vi "ReadKeithley6485Configuration.vi"(8 "Error In":errorcluster, 11 "ABLE Config File Ref In":T2) -> (0 "Error Out":errorcluster, 2 "Keithley 6485 Configuration":T1, 3 "ABLE Config File Ref Out":T2)   [LabVIEW 2012]
uses:
  <vilib>/Utility/config.llb/Config Data RefNum.ctl
  Keithley6485Configuration.ctl
  <vilib>/Utility/config.llb/Read Key (String).vi
  <vilib>/Utility/config.llb/NI_LVConfig.lvlib
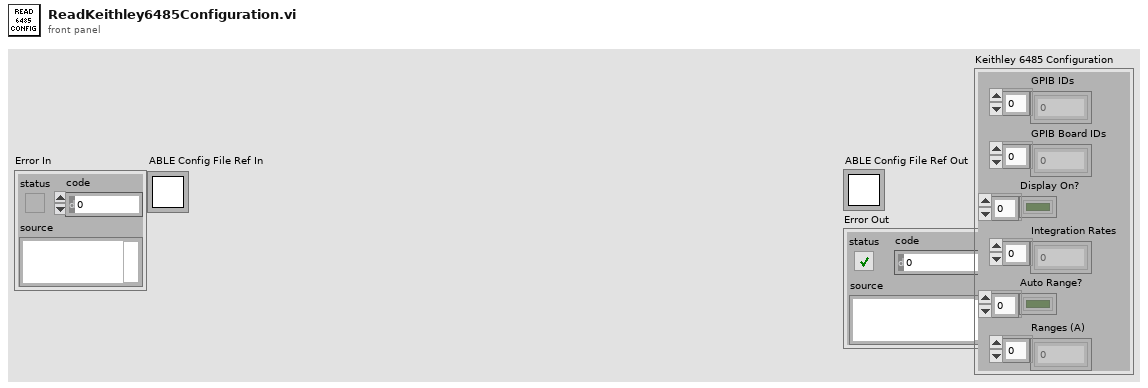
[diagram p1: front panel]
types:
  T1 = typedef "Keithley6485Configuration.ctl" = cluster{"GPIB IDs":u8[], "GPIB Board IDs":u8[], "Display On?":bool[], "Integration Rates":dbl[], "Auto Range?":bool[], "Ranges (A)":dbl[]}
  T2 = typedef "NI_LVConfig.lvlib/Config Data RefNum.ctl" = refnum<k1>
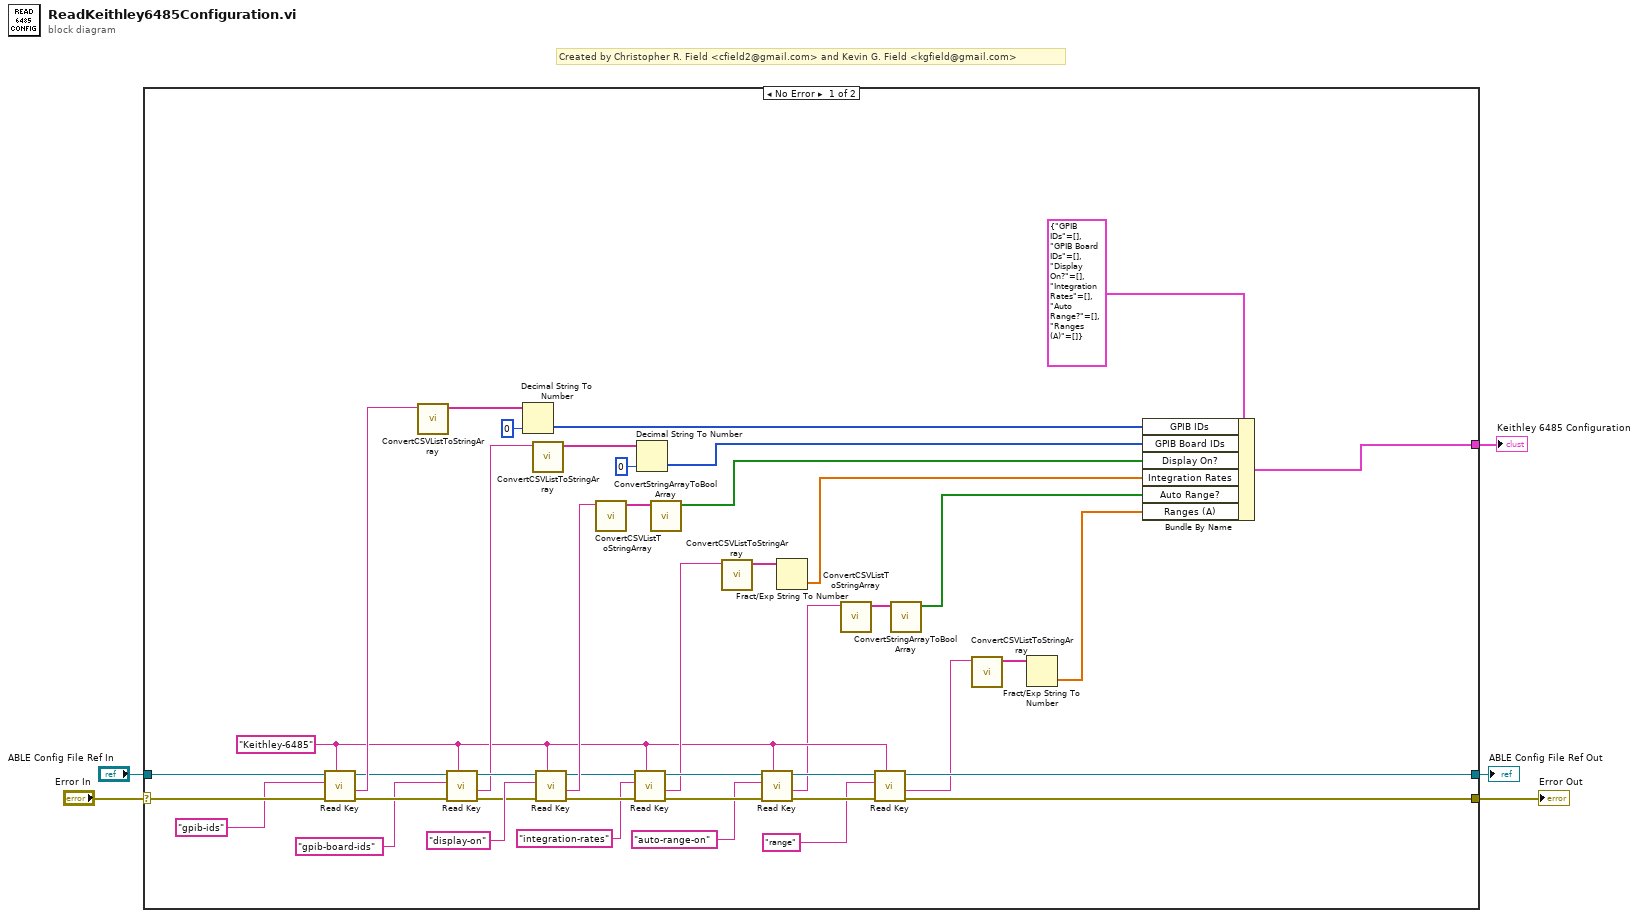
[diagram p0: block diagram]
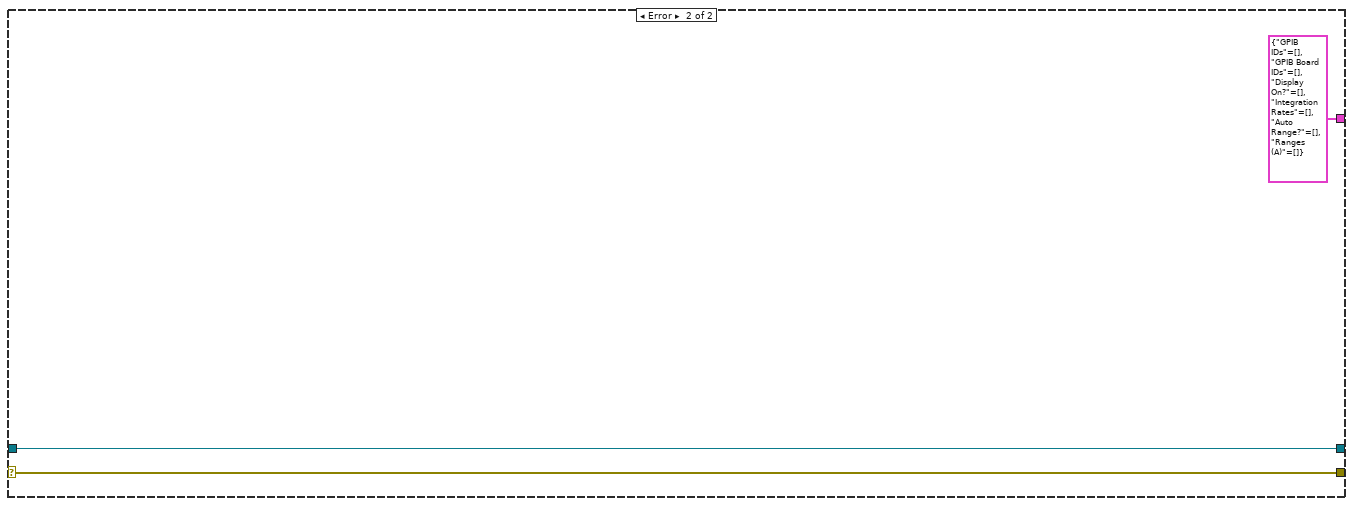
[diagram p2: hidden frame]
diagram:
  # "Created by Christopher R. Field <cfield2@gmail.com> and Kevin G. Field <kgfield@gmail.com>"
  n1 = case shown="No Error" "Error In" {
    selector: "Error In" -> [w48 w50]
    tunnel: "ABLE Config File Ref In" -> [w47 w51]
    tunnel: [w14 w51] -> w3
    tunnel: [w13 w50] -> w2
    tunnel: [w43 T1 {"GPIB IDs"=[], "GPIB Board IDs"=[], "Display On?"=[], "Integration Rates"=[], "Auto Range?"=[], "Ranges (A)"=[]} ("Keithley 6485 Configuration")] -> w1
    frame No Error {
      w10 = "Keithley-6485" ("section")
      n2 = call-poly <vilib>:"Read Key.vi"("section"=w10, "error in (no error)"=w48, "key"="gpib-ids", "refnum"=w47) -> ("error out"=w34:errorcluster, "value"=w42:string, "refnum out"=w37:T2)  [unwired: 4 in, 1 out]
      n3 = call "ConvertCSVListToStringArray.vi"("CSV List"=w42) -> ("String Array"=w41:string[])  [unwired: 10 in]
      n4 = call-poly <vilib>:"Read Key.vi"("section"=w10, "error in (no error)"=w34, "key"="gpib-board-ids", "refnum"=w37) -> ("error out"=w35:errorcluster, "value"=w31:string, "refnum out"=w36:T2)  [unwired: 4 in, 1 out]
      n5 = Decimal String To Number(string=w41, default (0L)=u8 0 ("default (0 I32)")) -> (number=w40:u8[])  [unwired: 1 in, 1 out]
      n6 = call "ConvertCSVListToStringArray.vi"("CSV List"=w31) -> ("String Array"=w32:string[])  [unwired: 10 in]
      n7 = call-poly <vilib>:"Read Key.vi"("section"=w10, "error in (no error)"=w35, "key"="display-on", "refnum"=w36) -> ("error out"=w19:errorcluster, "value"=w38:string, "refnum out"=w20:T2)  [unwired: 4 in, 1 out]
      n8 = call "ConvertCSVListToStringArray.vi"("CSV List"=w38) -> ("String Array"=w29:string[])  [unwired: 10 in]
      n9 = call-poly <vilib>:"Read Key.vi"("section"=w10, "error in (no error)"=w19, "key"="integration-rates", "refnum"=w20) -> ("error out"=w16:errorcluster, "value"=w12:string, "refnum out"=w18:T2)  [unwired: 4 in, 1 out]
      n10 = Decimal String To Number(string=w32, default (0L)=u8 0 ("default (0 I32)")) -> (number=w30:u8[])  [unwired: 1 in, 1 out]
      n11 = call "ConvertStringArrayToBoolArray.vi"("String Array"=w29) -> ("Boolean Array"=w28:bool[])  [unwired: 10 in]
      n12 = call "ConvertCSVListToStringArray.vi"("CSV List"=w12) -> ("String Array"=w26:string[])  [unwired: 10 in]
      n13 = call-poly <vilib>:"Read Key.vi"("section"=w10, "error in (no error)"=w16, "key"="auto-range-on", "refnum"=w18) -> ("error out"=w15:errorcluster, "value"=w9:string, "refnum out"=w17:T2)  [unwired: 4 in, 1 out]
      n14 = Fract/Exp String To Number(string=w26) -> (number=w25:dbl[])  [unwired: 3 in, 1 out]
      n15 = call "ConvertCSVListToStringArray.vi"("CSV List"=w9) -> ("String Array"=w24:string[])  [unwired: 10 in]
      n16 = call-poly <vilib>:"Read Key.vi"("section"=w10, "error in (no error)"=w15, "key"="range", "refnum"=w17) -> ("error out"=w13:errorcluster, "value"=w8:string, "refnum out"=w14:T2)  [unwired: 4 in, 1 out]
      n17 = call "ConvertStringArrayToBoolArray.vi"("String Array"=w24) -> ("Boolean Array"=w23:bool[])  [unwired: 10 in]
      n18 = call "ConvertCSVListToStringArray.vi"("CSV List"=w8) -> ("String Array"=w22:string[])  [unwired: 10 in]
      n19 = Fract/Exp String To Number(string=w22) -> (number=w21:dbl[])  [unwired: 3 in, 1 out]
      n20 = Bundle By Name(cluster=T1 {"GPIB IDs"=[], "GPIB Board IDs"=[], "Display On?"=[], "Integration Rates"=[], "Auto Range?"=[], "Ranges (A)"=[]} ("Keithley 6485 Configuration"), "GPIB IDs"=w40, "GPIB Board IDs"=w30, "Display On?"=w28, "Integration Rates"=w25, "Auto Range?"=w23, "Ranges (A)"=w21) -> (w43:T1)
    }
    frame Error {
    }
  }
  "ABLE Config File Ref Out" <- w3
  "Error Out" <- w2
  "Keithley 6485 Configuration" <- w1
